vi "Read settings.vi"(8 "error in (no error)":errorcluster, 9 "force loading?":bool=TRUE, 10 "settings name":string, 11 "ServiceManager in":refnum<class "ServiceManager.lvclass">) -> (0 "error out":errorcluster, 2 "setting name":string, 3 "ServiceManager out":refnum<class "ServiceManager.lvclass">)   [LabVIEW 2012, in "ServiceManager.lvclass"]
uses:
  ServiceManager.lvclass
  Murmex/LabVIEW/Murmex/Murmex/Murmex.lvclass
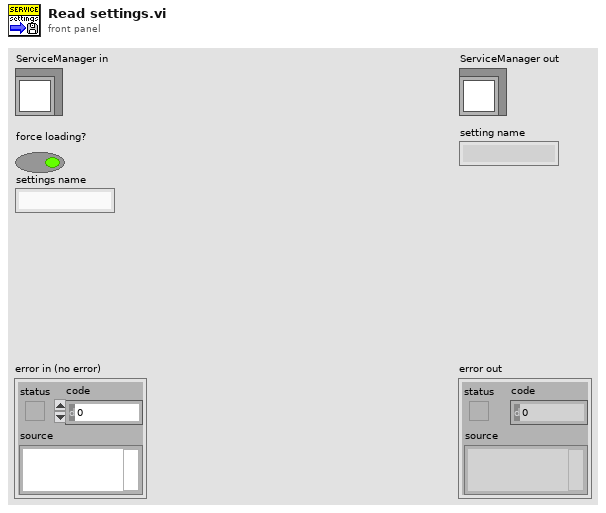
[diagram p1: front panel]
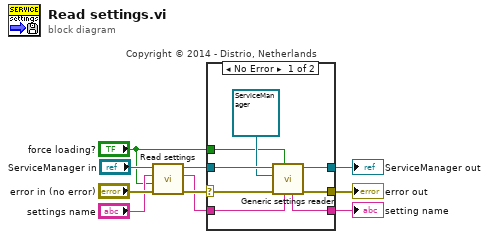
[diagram p0: block diagram]
diagram:
  n1 = call-parent "Read settings.vi"("error in (no error)"="error in (no error)", "force loading?"="force loading?", "settings name"="settings name", "Murmex in"="ServiceManager in") -> ("error out"=w7:errorcluster, "setting name"=w5:string, "Murmex out"=w3:refnum<class "ServiceManager.lvclass">)  [unwired: 5 in]
  n2 = case "Copyright © 2014 - Distrio, Netherlands" shown="No Error" w7 {
    selector: w7 -> [w18 w20]
    tunnel: [w12 w20] -> w6
    tunnel: [w17 w19] -> w2
    tunnel: w3 -> [w16 w19]
    tunnel: [w15 _] -> w4
    tunnel: w5 -> [w14 _]
    tunnel: "force loading?" -> [w11 _]
    frame No Error {
      n3 = call "Generic settings reader.vi"("settings name"=w14, "force loading?"=w11, "error in (no error)"=w18, "inheritance level"=refnum<class "ServiceManager.lvclass"> refnum ("ServiceManager.lvclass"), "Murmex in"=w16) -> ("error out"=w12:errorcluster, "Murmex out"=w17:refnum<class "ServiceManager.lvclass">, "setting name"=w15:string)  [unwired: 4 in]
    }
    frame Error {
    }
  }
  "error out" <- w6
  "ServiceManager out" <- w2
  "setting name" <- w4
